vi "仿真容器.vi"() -> ()   [LabVIEW 2010]
uses:
  液位全局变量.vi
panel:
  in  "泄漏量":dbl(slide)=0.9420289855072465 scale=0.0..10.0
  out "仿真容器":dbl(slide) scale=0.0..10.0
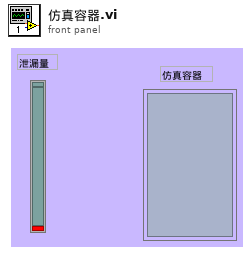
[diagram p1: front panel]
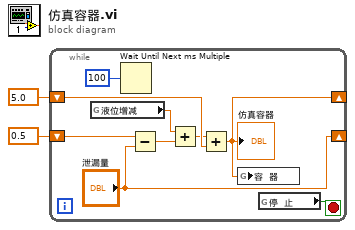
[diagram p0: block diagram]
diagram:
  n1 = while {
    shift-right: ["泄漏量"] -> _
    shift-left: 0.5 ("泄漏量") -> [w4]
    shift-right: [w10] -> _
    shift-left: 5.0 -> [w11]
    stop <- w9 stop-if-true
    n2 = global read "液位全局变量.vi" "液位增减"() -> (w7:dbl)
    n3 = Wait Until Next ms Multiple(millisecond multiple=u32 100) -> ()  [unwired: 1 out]
    n4 = Subtract(x=w4, y="泄漏量") -> (x-y=w6:dbl)
    n5 = Add(x=w7, y=w6) -> (x+y=w5:dbl)
    n6 = Add(x=w5, y=w11) -> (x+y=w10:dbl)
    "仿真容器" <- w10
    n7 = global write "液位全局变量.vi" "容  器"(w10) -> ()
    n8 = global read "液位全局变量.vi" "停  止"() -> (w9:bool)
  }
